vi "testSubdirectories - forward slash.vi"(8 "error in (no error)":errorcluster, 11 "TestCase in":refnum<class "Working Path Expansion Tests.lvclass">) -> (0 "error out":errorcluster, 3 "TestCase out":refnum<class "Working Path Expansion Tests.lvclass">)   [LabVIEW 2011, in "Working Path Expansion Tests.lvclass"]
uses:
  Working Path Expansion Tests.lvclass
  <vilib>/addons/_JKI Toolkits/VI Tester/TestCase.llb/TestCase.lvclass
  CLI Class/CLI.lvclass
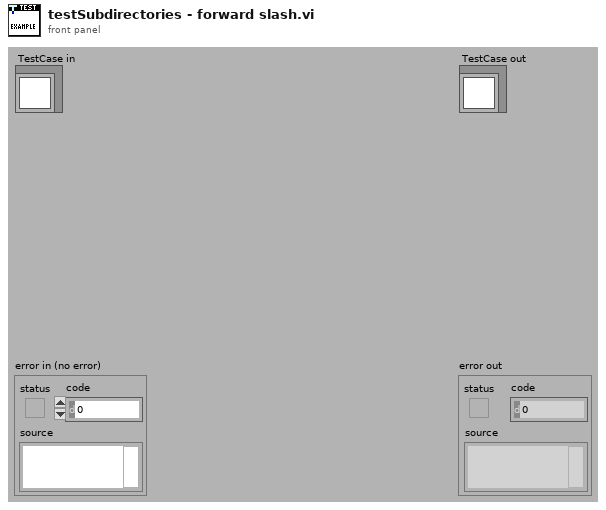
[diagram p1: front panel]
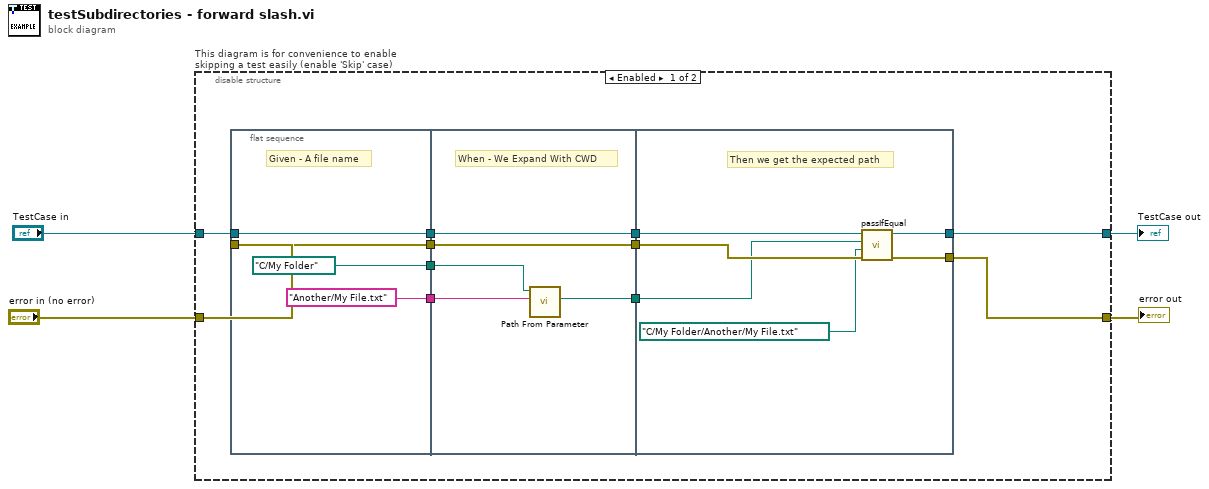
[diagram p0: block diagram]
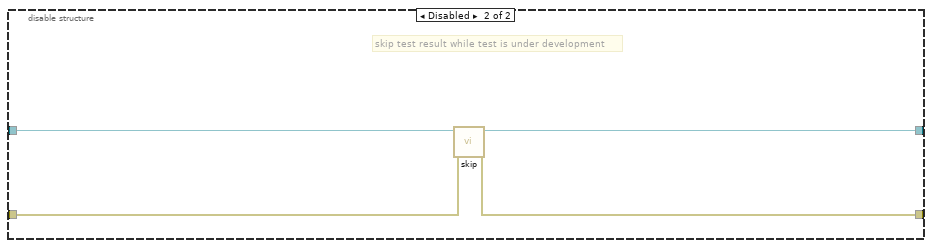
[diagram p2: hidden frame]
diagram:
  n1 = disable-structure "This diagram is for convenience to enable skipping a test easily (enable 'Skip' case)" shown="Enabled" {
    disable-tunnel: "TestCase in" -> [w13 w34]
    disable-tunnel: [w10 w32] -> w1
    disable-tunnel: [w9 w33] -> w3
    disable-tunnel: "error in (no error)" -> [w6 w31]
    frame Enabled {
      n2 = flat-sequence {
        tunnel: [path "C:/My Folder" ("Working Directory")] -> w15
        tunnel: ["Another/My File.txt"] -> w14
        tunnel: w13 -> [w17]
        tunnel: [w17] -> w12
        tunnel: [w16] -> w7
        tunnel: w6 -> [w16]
        tunnel: w15 -> [w24]
        tunnel: w14 -> [w23]
        tunnel: w12 -> [w22]
        tunnel: [w22] -> w11
        tunnel: [w21] -> w8
        tunnel: w7 -> [w21]
        tunnel: [w20] -> w5
        tunnel: w11 -> [w30]
        tunnel: [w29] -> w10
        tunnel: [w28] -> w9
        tunnel: w8 -> [w27]
        tunnel: w5 -> [w26]
        frame #0 {
          # "Given - A file name"
        }
        frame #1 {
          # "When - We Expand With CWD"
          n3 = call "Path From Parameter.vi"("Path Parameter"=w23, "Working Directory"=w24) -> ("Full Path"=w20:path)  [unwired: 9 in]
        }
        frame #2 {
          # "Then we get the expected path"
          n4 = call-dynamic "passIfEqual.vi"("error in (no error)"=w27, "y"=path "C:/My Folder/Another/My File.txt" ("Working Directory"), "x"=w26, "TestCase in"=w30) -> ("error out"=w28:errorcluster, "TestCase out"=w29:refnum<class "Working Path Expansion Tests.lvclass">)  [unwired: 6 in]
        }
      }
    }
    frame Disabled {
      # "skip test result while test is under development"
      n5 = call <vilib>:"skip.vi"("error in (no error)"=w31, "TestCase in"=w34) -> ("error out"=w33:errorcluster, "TestCase out"=w32:refnum<class "Working Path Expansion Tests.lvclass">)  [unwired: 8 in]
    }
  }
  "error out" <- w3
  "TestCase out" <- w1
